vi "QTrkQueueImageU16.vi"(0 "QTrk Instance":T1, 2 "Timestamp":i32, 4 "frame#":i32, 5 "error in (no error)":errorcluster, 6 "zlutPlane":i32, 7 "zlutIndex":i32, 9 "Image (U16)":u16[][](array[numeric])) -> (14 "QTrk Instance":T1, 19 "error out":errorcluster)   [LabVIEW 2011]
uses:
  QTrkInstance.ctl
  QTrkLocalizationJob.ctl
  XYZf.ctl
  QTrkDLL.vi
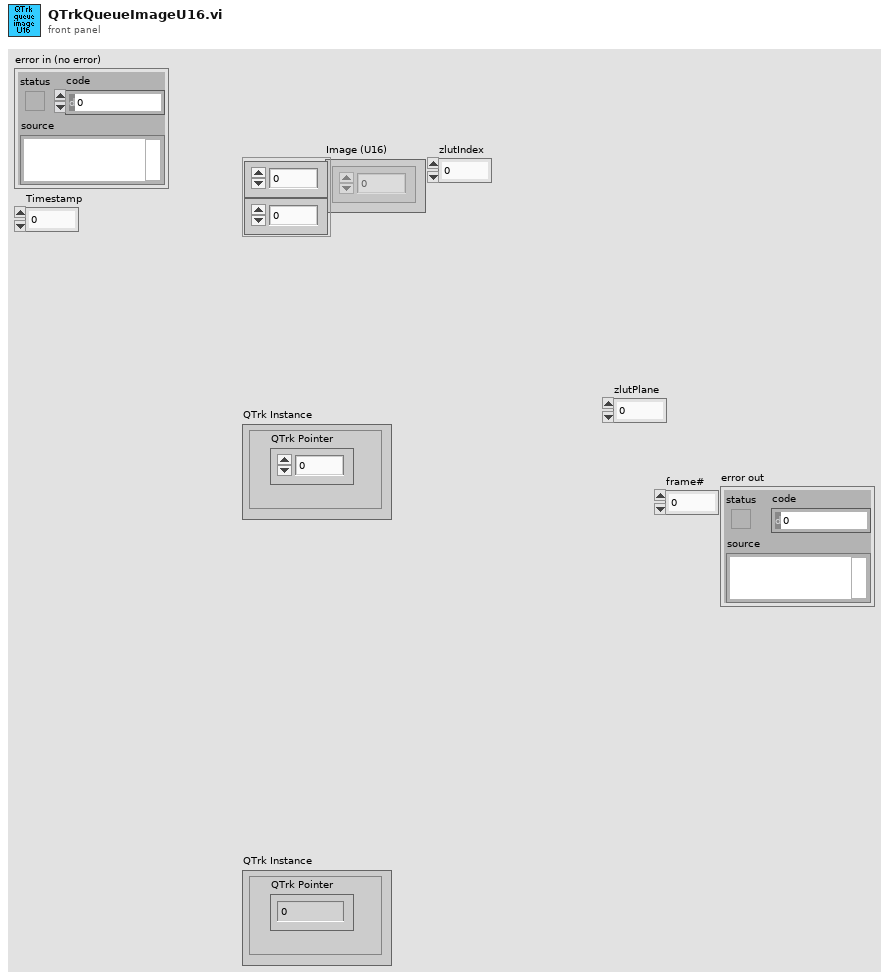
[diagram p1: front panel]
types:
  T1 = typedef "QTrkInstance.ctl" = cluster{"QTrk Pointer":u64}
  T2 = typedef "QTrkLocalizationJob.ctl" = cluster{"Frame#":u32, "Timestamp":u32, "ZLUT Index / bead#":i32, "ZLUT Plane":i32, "Initial guess":T3}
  T3 = typedef "XYZf.ctl" = cluster{"X":sgl, "Y":sgl, "Z":sgl}
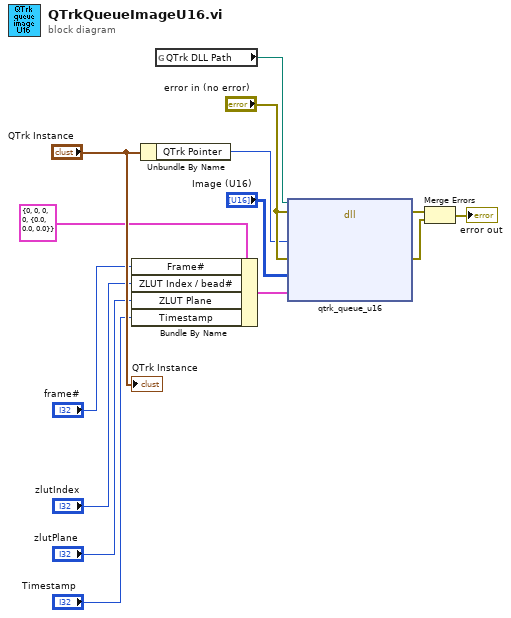
[diagram p0: block diagram]
diagram:
  n1 = Bundle By Name(cluster=T2 {"Frame#"=0, "Timestamp"=0, "ZLUT Index / bead#"=0, "ZLUT Plane"=0, "Initial guess"={"X"=0.0, "Y"=0.0, "Z"=0.0}} ("Queue Params"), "Frame#"="frame#", "ZLUT Index / bead#"="zlutIndex", "ZLUT Plane"="zlutPlane", "Timestamp"="Timestamp") -> (w13:T2)
  n2 = Unbundle By Name("QTrk Instance") -> ("QTrk Pointer"=w3:u64)
  n3 = global read "QTrkDLL.vi" "QTrk DLL Path"() -> (w2:path)
  n4 = dll-call lib="D:/jcnossen1/cudaqi-tracker/bin/jtrk-labview.dll" fn="qtrk_queue_u16"(path in=w2, error in="error in (no error)", "tracker"=w3, "error"="error in (no error)", "data"="Image (U16)", "params"=w13) -> (error out=w6:errorcluster, "error"=w5:errorcluster)  [unwired: 5 in, 1 out]
  n5 = Merge Errors(w6, w5) -> (→"error out":errorcluster)
  "QTrk Instance" <- "QTrk Instance"
